vi "Assignment5_PeopleCounter.vi"() -> ()   [LabVIEW 2024]
panel:
  out "Number of people":dbl
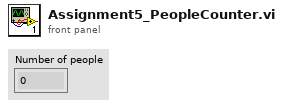
[diagram p1: front panel]
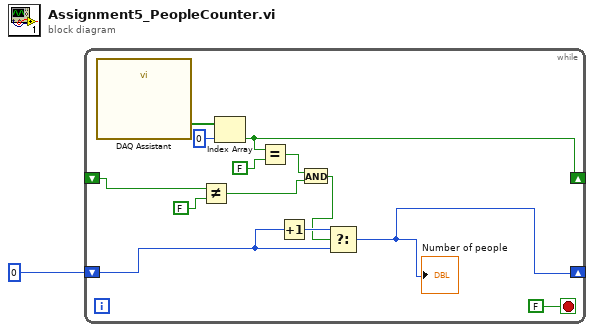
[diagram p0: block diagram]
diagram:
  n1 = while {
    shift-right: [w11] -> _
    shift-left: 0 -> [w12]
    shift-right: [w4] -> _
    shift-left: _ -> [w8]
    stop <- FALSE stop-if-true
    n2 = call "DAQ Assistant"() -> ("data"=w9:bool[])  [unwired: 17 in, 2 out]
    n3 = Not Equal?(x=w8, y=FALSE) -> (x != y?=w6:bool)
    n4 = Index Array(array=w9, index=0) -> (element=w4:bool)
    n5 = Equal?(x=w4, y=FALSE) -> (x = y?=w5:bool)
    n6 = Increment(x=w12) -> (x+1=w13:i32)
    n7 = And(x=w5, y=w6) -> (x .and. y?=w2:bool)
    n8 = Select(t=w13, s=w2, f=w12) -> (s? t:f=w11:i32)
    "Number of people" <- w11
  }
